vi "Write Fixed Header.vi"(10 "Fixed Header":u8 format="%08b", 11 "ControlPacket in":refnum<class "ControlPacket.lvclass">) -> (3 "ControlPacket out":refnum<class "ControlPacket.lvclass">)   [LabVIEW 2013, in "ControlPacket.lvclass"]
uses:
  ControlPacket.lvclass
  ControlPacket.lvclass/ControlPacket.ctl
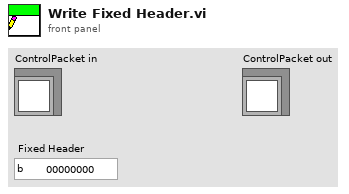
[diagram p1: front panel]
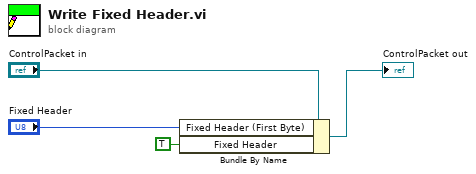
[diagram p0: block diagram]
diagram:
  n1 = Bundle By Name(cluster="ControlPacket in", "Fixed Header (First Byte)"="Fixed Header", "Fixed Header"=TRUE) -> (→"ControlPacket out":refnum<class "ControlPacket.lvclass">)
